vi "TOML to LabVIEW.vi"(7 "Default Value":variant, 8 "error in (no error)":errorcluster, 9 "Parent":string, 10 "Error if missing element":bool caption="Error if missing element (F)", 11 "TOML Value":T1) -> (0 "error out":errorcluster, 2 "Missing elements":string[](array[string]), 3 "LV Value":variant)   [LabVIEW 2020, in "TOML.lvlib"]
doc: "Extract variables from TOML data as defined by the \"Default value\" input\n\n<b>By default</b> the behaviour is that if an element is not found (by label) in the TOML data, the default value as defined by the input will be returned.\n<b>If on the other hand</b> you want this VI to return an error when an element is not found, set \"Error if missing element\" so <b>True</b>"
uses:
  TOML.lvlib
  TOML Value.ctl
  Value.ctl
  Value Type.ctl
  Key-Value Pair.ctl
  <vilib>/ErrorRing/Error Ring.xnode
  <vilib>/Utility/Data Type/NI_Data Type.lvlib
  <vilib>/JDP Science/JDP Science Common Utilities/JDP Utility.lvlib
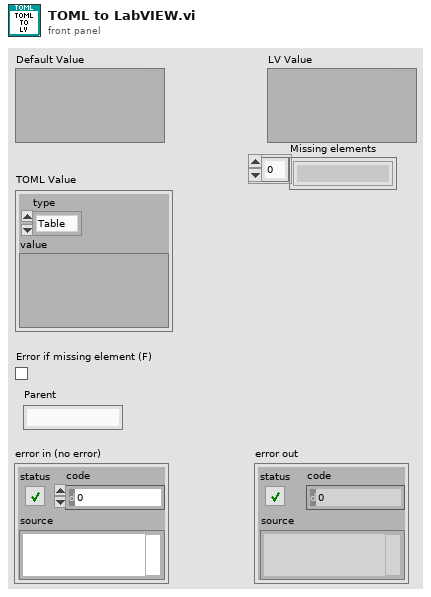
[diagram p1: front panel]
types:
  T1 = typedef "TOML.lvlib/TOML Value.ctl" = cluster{"type":enum16{"Table", "Array", "String", "Integer", "Float", "Boolean", "Offset Date-Time", "Local Date-Time", "Local Date", "Local Time", "Path"}, "value":variant}
  T2 = typedef "TOML.lvlib/Value.ctl" = cluster{"Type":T3, "Value":variant}
  T3 = typedef "TOML.lvlib/Value Type.ctl" = enum16{"Table", "Array", "String", "Integer", "Float", "Boolean", "Offset Date-Time", "Local Date-Time", "Local Date", "Local Time", "Path"}
  T4 = typedef "TOML.lvlib/Key-Value Pair.ctl" = cluster{"Key":string, "Value":T2}
  T5 = typedef "NI_Data Type.lvlib/Data Type.ctl" = enum8{"Invalid Type", "Void", "I8", "I16", "I32", "I64", "U8", "U16", "U32", "U64", "Single Float", "Double Float", "Extended Float", "Single Complex", "Double Complex", "Extended Complex", "Enum U8", "Enum U16", "Enum U32", "Enum U64", "Single Float With Unit", "Double Float With Unit", "Extended Float With Unit", "Single Complex with Unit", "Double Complex with Unit", "Extended Complex with Unit", "Boolean", "String", "Path", "Picture", "Tag", "Array", "Cluster", "Variant", "LV Variant", "Waveform", "Timestamp", "Digital Waveform", "Digital Data", "ExpressData", "Refnum", "External Data", "VI", "Poly VI", "LabVIEW Class Instance", "Fixed Point", "Set Collection", "Map Collection"}
  T6 = typedef "NI_Data Type.lvlib/Memory Info.ctl" = cluster{"Type":T7, "Size":u32}
  T7 = typedef "NI_Data Type.lvlib/Memory Type.ctl" = enum16{"Variable", "Fixed", "Bounded"}
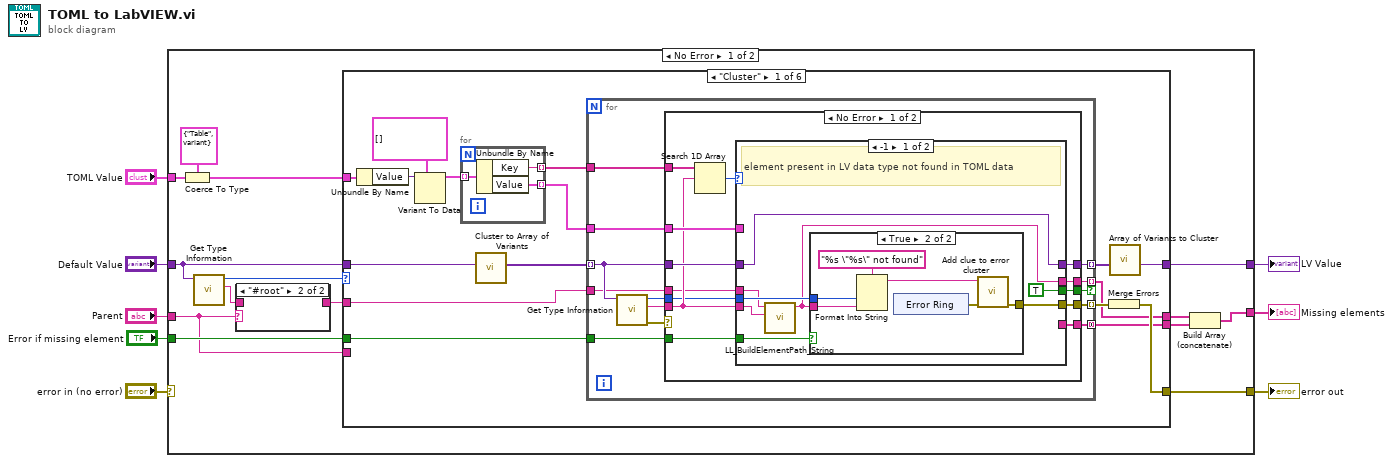
[diagram p0: block diagram]
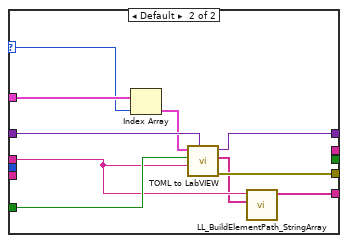
[diagram p4: hidden frame]
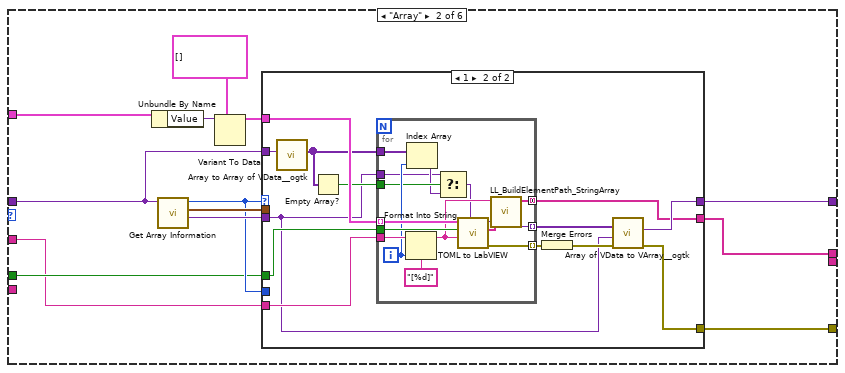
[diagram p6: hidden frame]
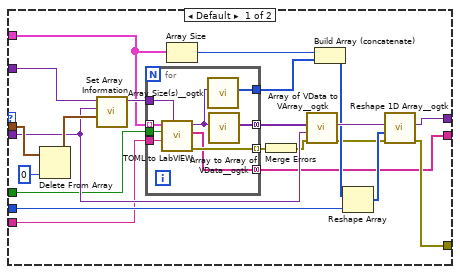
[diagram p7: hidden frame]
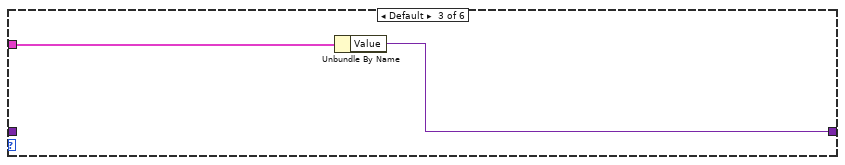
[diagram p8: hidden frame]
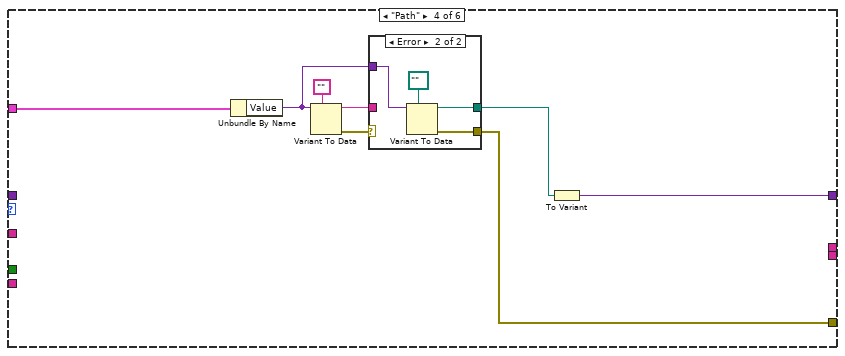
[diagram p9: hidden frame]
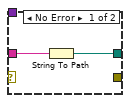
[diagram p10: hidden frame]
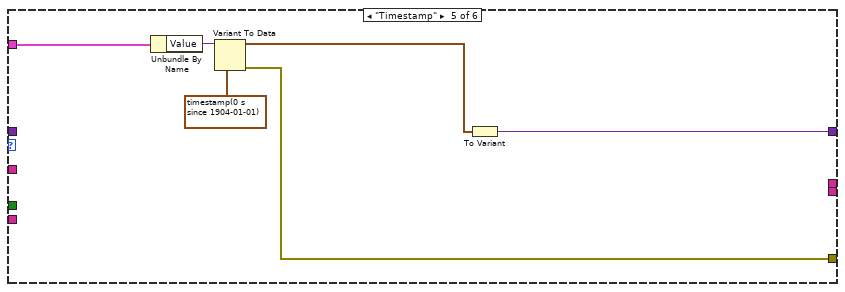
[diagram p11: hidden frame]
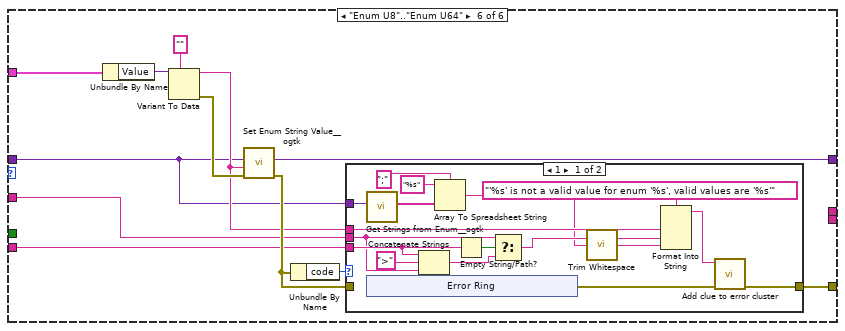
[diagram p12: hidden frame]
diagram:
  n1 = case shown="No Error" "error in (no error)" {
    selector: "error in (no error)" -> [_ w221]
    tunnel: "Default Value" -> [w11 _]
    tunnel: [w21 _] -> w7
    tunnel: "TOML Value" -> [w20 _]
    tunnel: [w10 w221] -> w4
    tunnel: "Error if missing element" -> [w17 _]
    tunnel: [w14 _] -> w2
    tunnel: "Parent" -> [w9 _]
    frame No Error {
      n2 = Coerce To Type(0:w20, 1:T2 {"Type"=enum."Table", "Value"=variant} ("type")) -> (2:w19:T2)
      n3 = call <vilib>:"Get Type Information.vi"("variant"=w11) -> ("name"=w13:string, "type"=w22:T5)  [unwired: 6 in, 3 out]
      n4 = case shown="\"#root\"" w9 {
        tunnel: [w23 _] -> w12
        tunnel: w13 -> [w23 _]
        frame Default {
        }
        frame "#root" {
        }
      }
      n5 = case shown="\"Cluster\"" w22 {
        tunnel: w19 -> [w39 w108 w169 w177 w189 w201]
        tunnel: w11 -> [w31 w104 _ _ _ w190]
        tunnel: [w28 w101 w168 w175 w187 w198] -> w21
        tunnel: [w32 w99 _ w170 w185 w194] -> w10
        tunnel: w12 -> [w24 w97 _ _ _ w192]
        tunnel: w17 -> [w27 w98 _ _ _ _]
        tunnel: [w26 w96 _ _ _ _] -> w16
        tunnel: [w25 _ _ _ _ _] -> w15
        tunnel: w9 -> [_ _ _ _ _ w191]
        frame "Cluster" {
          n6 = Unbundle By Name(w39) -> ("Value"=w38:variant)
          n7 = Variant To Data(type=T4[] [], Variant=w38) -> (data=w35:T4[])  [unwired: 1 in, 1 out]
          n8 = for {
            tunnel: w35 -> [w40] mode=indexing
            tunnel: [w42] -> w36 mode=indexing
            tunnel: [w41] -> w34 mode=indexing
            n9 = Unbundle By Name(w40) -> ("Key"=w42:string, "Value"=w41:T2)
          }
          n10 = call <vilib>:"Cluster to Array of Variants.vi"("Cluster"=w31) -> ("Array of Cluster Elements"=w30:variant[])  [unwired: 10 in]
          n11 = for {
            tunnel: w30 -> [w53] mode=indexing
            tunnel: w36 -> [w55]
            tunnel: w34 -> [w54]
            tunnel: [w52] -> w33 mode=indexing
            tunnel: [w51] -> w29 mode=indexing
            tunnel: w27 -> [w47]
            tunnel: [w46] -> w26 mode=indexing if=w45
            tunnel: [w44] -> w25 mode=concatenating
            tunnel: w24 -> [w43]
            n12 = call <vilib>:"Get Type Information.vi"("variant"=w53) -> ("error out"=w48:errorcluster, "name"=w50:string, "type"=w49:T5)  [unwired: 6 in, 2 out]
            n13 = case shown="No Error" w48 {
              selector: w48 -> [_ w95]
              tunnel: w55 -> [w68 _]
              tunnel: w54 -> [w67 _]
              tunnel: w53 -> [w66 w94]
              tunnel: [w64 w95] -> w52
              tunnel: [w63 w94] -> w51
              tunnel: w50 -> [w62 _]
              tunnel: w49 -> [w61 _]
              tunnel: w47 -> [w60 _]
              tunnel: [w59 _] -> w46
              tunnel: [w58 _] -> w45
              tunnel: w43 -> [w57 _]
              tunnel: [w56 _] -> w44
              frame No Error {
                n14 = Search 1D Array(1D array=w68, element=w62) -> (index of element=w65:i32)  [unwired: 1 in]
                n15 = case shown="-1" w65 {
                  selector: w65 -> [_ w88]
                  tunnel: w67 -> [_ w93]
                  tunnel: w66 -> [w73 w92]
                  tunnel: [w75 w89] -> w64
                  tunnel: [w73 w90] -> w63
                  tunnel: w62 -> [w72 _]
                  tunnel: w61 -> [w76 _]
                  tunnel: w60 -> [w74 w87]
                  tunnel: [w69 _] -> w59
                  tunnel: [TRUE _] -> w58
                  tunnel: w57 -> [w71 w86]
                  tunnel: [_ w84] -> w56
                  frame -1 {
                    # "element present in LV data type not found in TOML data"
                    n16 = call "LL_BuildElementPath_String.vi"("Name"=w72, "parent Name"=w71) -> ("full name"=w69:string)  [unwired: 9 in]
                    n17 = case shown="True" w74 {
                      tunnel: w69 -> [_ w82]
                      tunnel: w76 -> [_ w81]
                      tunnel: [_ w79] -> w75
                      frame False {
                      }
                      frame True {
                        n18 = Format Into String(format string="%s \"%s\" not found", w81, w82) -> (resulting string=w77:string)  [unwired: 2 in, 1 out]
                        n19 = xnode "Error Ring"() -> ("error out"=w78:errorcluster)
                        n20 = call "Add clue to error cluster.vi"("error in (no error)"=w78, "String"=w77) -> ("error out"=w79:errorcluster)  [unwired: 9 in]
                      }
                    }
                  }
                  frame Default {
                    n21 = Index Array(array=w93, index=w88) -> (element=w91:T2)
                    n22 = call "TOML to LabVIEW.vi"("Default Value"=w92, "Parent"=w86, "Error if missing element"=w87, "TOML Value"=w91) -> ("error out"=w89:errorcluster, "Missing elements"=w85:string[], "LV Value"=w90:variant)  [unwired: 5 in]
                    n23 = call "LL_BuildElementPath_StringArray.vi"("Names"=w85, "parent Name"=w86) -> ("full name"=w84:string[])  [unwired: 9 in]
                  }
                }
              }
              frame Error {
              }
            }
          }
          n24 = Merge Errors(w33) -> (w32:errorcluster)
          n25 = call <vilib>:"Array of Variants to Cluster.vi"("Array of Variants"=w29) -> ("Cluster of Variants"=w28:variant)  [unwired: 10 in]
        }
        frame "Array" {
          n26 = Unbundle By Name(w108) -> ("Value"=w107:variant)
          n27 = call <vilib>:"Get Array Information.vi"("variant"=w104) -> ("array element data type"=w105:variant, "array lengths"=w103:T6[], "number of dimensions"=w100:i32)  [unwired: 7 in, 1 out]
          n28 = Variant To Data(type=T2[] [], Variant=w107) -> (data=w102:T2[])  [unwired: 1 in, 1 out]
          n29 = case shown="1" w100 {
            tunnel: w105 -> [w119 w140]
            tunnel: w104 -> [w130 w144]
            tunnel: w103 -> [w129 _]
            tunnel: w102 -> [w125 w152]
            tunnel: [w122 w150] -> w101
            tunnel: w100 -> [w118 _]
            tunnel: [w112 w148] -> w99
            tunnel: w98 -> [w111 w147]
            tunnel: [w110 w145] -> w96
            tunnel: w97 -> [w109 w146]
            frame Default {
              n30 = Delete From Array(array=w129, index=0) -> (array with subset deleted=w127:T6[])  [unwired: 1 in, 1 out]
              n31 = call <vilib>:"Set Array Information.vi"("Array Lengths"=w127, "Array Element"=w119, "Variant in"=w130) -> ("Variant out"=w126:variant)  [unwired: 7 in, 1 out]
              n32 = for {
                tunnel: w126 -> [w139]
                tunnel: w125 -> [w136] mode=indexing
                tunnel: [w138] -> w123
                tunnel: [w137] -> w121 mode=concatenating
                tunnel: [w134] -> w115 mode=indexing
                tunnel: w111 -> [w133]
                tunnel: [w132] -> w110 mode=concatenating
                tunnel: w109 -> [w131]
                n33 = call "TOML to LabVIEW.vi"("Default Value"=w139, "Parent"=w131, "Error if missing element"=w133, "TOML Value"=w136) -> ("error out"=w134:errorcluster, "Missing elements"=w132:string[], "LV Value"=w135:variant)  [unwired: 5 in]
                n34 = call <userlib>:"Array Size(s)__ogtk.vi"("Array"=w135) -> ("Size(s)"=w138:u32[])  [unwired: 8 in, 2 out]
                n35 = call <userlib>:"Array to Array of VData__ogtk.vi"("MultiD Array"=w135) -> ("1D Array of Variants"=w137:variant[])  [unwired: 9 in, 1 out]
              }
              n36 = Array Size(array=w125) -> (size(s)=w124:i32)
              n37 = Merge Errors(w115) -> (w114:errorcluster)
              n38 = call <userlib>:"Array of VData to VArray__ogtk.vi"("error in (no error)"=w114, "Element Type (when empty)"=w119, "1D Array of VData"=w121) -> ("error out"=w113:errorcluster, "VArray"=w120:variant)  [unwired: 7 in]
              n39 = Build Array (concatenate)(w124, w123) -> (w117:u32[])
              n40 = Reshape Array(w117, w118) -> (w116:u32[])
              n41 = call <userlib>:"Reshape 1D Array__ogtk.vi"("error in (no error)"=w113, "Size(s)"=w116, "1D Array"=w120) -> ("error out"=w112:errorcluster, "Reshaped VArray"=w122:variant)  [unwired: 7 in]
            }
            frame 1 {
              n42 = call <userlib>:"Array to Array of VData__ogtk.vi"("MultiD Array"=w144) -> ("1D Array of Variants"=w142:variant[])  [unwired: 9 in, 1 out]
              n43 = Empty Array?(array=w142) -> (empty?=w141:bool)
              n44 = for {
                tunnel: w152 -> [w167] mode=indexing
                tunnel: [w166] -> w151 mode=indexing
                tunnel: [w165] -> w143 mode=indexing
                tunnel: w147 -> [w164]
                tunnel: [w159] -> w145 mode=concatenating
                tunnel: w146 -> [w162]
                tunnel: w142 -> [w158]
                tunnel: w141 -> [w156]
                tunnel: w140 -> [w153]
                i -> [w157]
                n45 = Format Into String(format string="[%d]", initial string=w162, w157) -> (resulting string=w161:string)  [unwired: 1 in, 1 out]
                n46 = Index Array(array=w158, index=w157) -> (element=w155:variant)
                n47 = Select(t=w153, s=w156, f=w155) -> (s? t:f=w154:variant)
                n48 = call "TOML to LabVIEW.vi"("Default Value"=w154, "Parent"=w161, "Error if missing element"=w164, "TOML Value"=w167) -> ("error out"=w165:errorcluster, "Missing elements"=w160:string[], "LV Value"=w166:variant)  [unwired: 5 in]
                n49 = call "LL_BuildElementPath_StringArray.vi"("Names"=w160, "parent Name"=w161) -> ("full name"=w159:string[])  [unwired: 9 in]
              }
              n50 = Merge Errors(w143) -> (w149:errorcluster)
              n51 = call <userlib>:"Array of VData to VArray__ogtk.vi"("error in (no error)"=w149, "Element Type (when empty)"=w140, "1D Array of VData"=w151) -> ("error out"=w148:errorcluster, "VArray"=w150:variant)  [unwired: 7 in]
            }
          }
        }
        frame Default {
          n52 = Unbundle By Name(w169) -> ("Value"=w168:variant)
        }
        frame "Path" {
          n53 = Unbundle By Name(w177) -> ("Value"=w173:variant)
          n54 = Variant To Data(type="", Variant=w173) -> (data=w172:string, error out=w174:errorcluster)  [unwired: 1 in]
          n55 = case shown="Error" w174 {
            tunnel: w173 -> [_ w183]
            tunnel: w172 -> [w179 _]
            tunnel: [w178 w181] -> w171
            tunnel: [_ w180] -> w170
            frame No Error {
              n56 = String To Path(string=w179) -> (path=w178:path)
            }
            frame Error {
              n57 = Variant To Data(type=path "" ("path"), Variant=w183) -> (data=w181:path, error out=w180:errorcluster)  [unwired: 1 in]
            }
          }
          n58 = To Variant(anything=w171) -> (Variant=w175:variant)
        }
        frame "Timestamp" {
          n59 = Unbundle By Name(w189) -> ("Value"=w188:variant)
          n60 = Variant To Data(type=timestamp(0 s since 1904-01-01), Variant=w188) -> (data=w184:timestamp, error out=w185:errorcluster)  [unwired: 1 in]
          n61 = To Variant(anything=w184) -> (Variant=w187:variant)
        }
        frame "Enum U8".."Enum U64" {
          n62 = Unbundle By Name(w201) -> ("Value"=w200:variant)
          n63 = Variant To Data(type="", Variant=w200) -> (data=w193:string, error out=w197:errorcluster)  [unwired: 1 in]
          n64 = call <userlib>:"Set Enum String Value__ogtk.vi"("error in (no error)"=w197, "String Value"=w193, "Default Enum Value"=w190) -> ("error out"=w195:errorcluster, "Enum"=w198:variant)  [unwired: 7 in]
          n65 = Unbundle By Name(w195) -> ("code"=w196:i32)
          n66 = case shown="1" w196 {
            tunnel: [w218 w220] -> w194
            tunnel: w195 -> [_ w220]
            tunnel: w193 -> [w211 _]
            tunnel: w192 -> [w203 _]
            tunnel: w191 -> [w212 _]
            tunnel: w190 -> [w208 _]
            frame 1 {
              n67 = call <userlib>:"Get Strings from Enum__ogtk.vi"("Enum"=w208) -> ("Enum Strings"=w207:string[])  [unwired: 7 in, 3 out]
              n68 = xnode "Error Ring"() -> ("error out"=w217:errorcluster)
              n69 = Concatenate Strings(w212, ">", w203) -> (w209:string)
              n70 = Array To Spreadsheet String(delimiter (Tab)=";" ("format string"), array=w207, 3:"%s" ("format string")) -> (spreadsheet string=w206:string)
              n71 = Empty String/Path?(string/path=w212) -> (empty?=w214:bool)
              n72 = Select(t=w203, s=w214, f=w209) -> (s? t:f=w213:string)
              n73 = call <vilib>:"Trim Whitespace.vi"("string"=w206) -> ("trimmed string"=w202:string)  [unwired: 1 in]
              n74 = Format Into String(format string="'%s' is not a valid value for enum '%s', valid values are '%s'", w211, w213, w202) -> (resulting string=w216:string)  [unwired: 2 in, 1 out]
              n75 = call "Add clue to error cluster.vi"("error in (no error)"=w217, "String"=w216) -> ("error out"=w218:errorcluster)  [unwired: 9 in]
            }
            frame Default {
            }
          }
        }
      }
      n76 = Build Array (concatenate)(w16, w15) -> (w14:string[])
    }
    frame Error {
    }
  }
  "LV Value" <- w7
  "error out" <- w4
  "Missing elements" <- w2
